vi "485 comm RT Driver VI.vi"(6 "Device Clock":string, 9 "Device Inputs FIFO":refnum<k33>, 10 "Device Outputs FIFO":refnum<k33>, 11 "Device Reference":T1 format="%.0x") -> ()   [LabVIEW 2015, in "485 comm Custom Device.lvlib"]
uses:
  485 comm Custom Device.lvlib
  <vilib>/NI Veristand/Custom Device API/Custom Device Item Ref.ctl
  <vilib>/NI Veristand/Custom Device API/Custom Device Channel Type.ctl
  Serial - Settings.ctl
  <vilib>/NI Veristand/Custom Device API/Message Response (String).ctl
  <vilib>/NI Veristand/Custom Device API/Message Response (Byte Array).ctl
  <vilib>/NI Veristand/Custom Device API/Get Item Property (Variant).vi
  <vilib>/NI Veristand/Custom Device API/Get Item Property (String).vi
  <vilib>/NI Veristand/Custom Device API/Get Item Property (U16).vi
  <vilib>/NI Veristand/Custom Device API/Get Item Property (U32).vi
  <vilib>/Instr/_visa.llb/VISA Configure Serial Port (Instr).vi
  <vilib>/NI Veristand/Custom Device API/Get Item Property (Boolean).vi
  <vilib>/NI Veristand/Custom Device API/Custom Device API.lvlib
  <vilib>/NI VeriStand/Custom Device Tools/Custom Device Utility Library/Custom Device Utility Library.lvlib
panel:
  in  "Initialization Status Notifier":refnum<notifier>
  in  "Status Notifier":refnum<notifier>
  # "Custom Device Template\nv1.0"
  # "Use this template as a starting point for creating a custom device code module. The input controls shown here are specially named controls that the system will use to provide the device loop with data. The controls are not required for the device loop to run. For instance, if the device doesn't produce any output data, then you don't need the Device Outputs FIFO control. If you do use these controls, however, they need to have these exact names to be functional."
  # "The optional status notifier element is used to notify the RT engine of the last state of the custom device, and to indicate the device has completed execution. If this control is not used, a default No Error value is returned to the system when the device finishes execution.\n\nNote: This error state is not checked until the system shuts down. Use an output status channel to send more immediate status values to the system."
  # "This optional input can be used to send the VeriStand Engine the final status of the custom device initalization process. If this control exists on the custom device front panel, the VeriStand Engine will wait for a status update before starting up. If the custom device reports an error, that will abort the execution of the current configuration in the VeriStand Engine.\n\nThis control can be deleted if the custom device does not need to send the initialization status update."
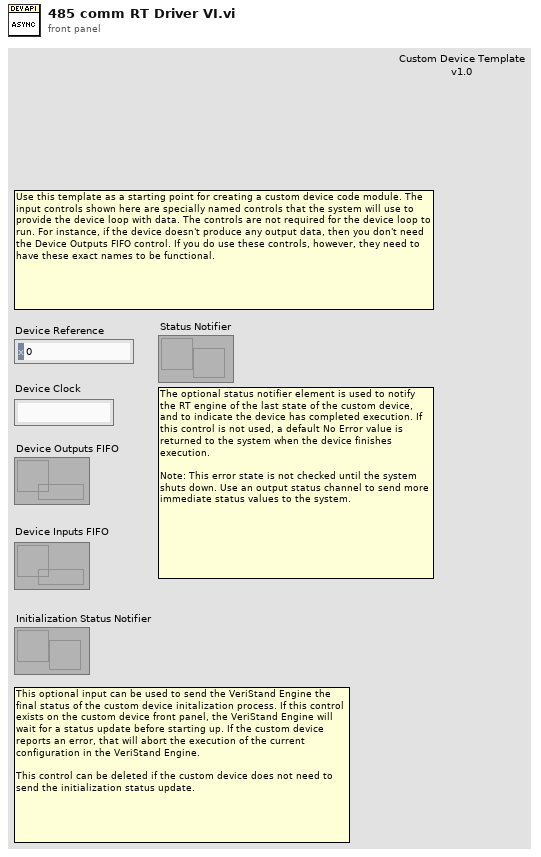
[diagram p1: front panel]
types:
  T1 = typedef "Custom Device API.lvlib/Custom Device Item Ref.ctl" = u64
  T2 = typedef "485 comm Custom Device.lvlib/Serial - Settings.ctl" = cluster{"baud rate":u32, "data bits":u16, "parity":enum16{"None", "Odd", "Even", "Mark", "Space"}, "stop bits":u16, "flow control":u16}
  T3 = typedef "Custom Device API.lvlib/Custom Device Channel Type.ctl" = enum16{"Input", "Output"}
  T4 = typedef "Custom Device API.lvlib/Custom Device Engine Event Ref.ctl" = refnum<event-registration>
  T5 = typedef "Custom Device API.lvlib/Message Response (String).ctl" = cluster{"Response":string, "Error":errorcluster}
  T6 = typedef "Custom Device API.lvlib/Message Response (Byte Array).ctl" = cluster{"Response":u8[], "Error":errorcluster}
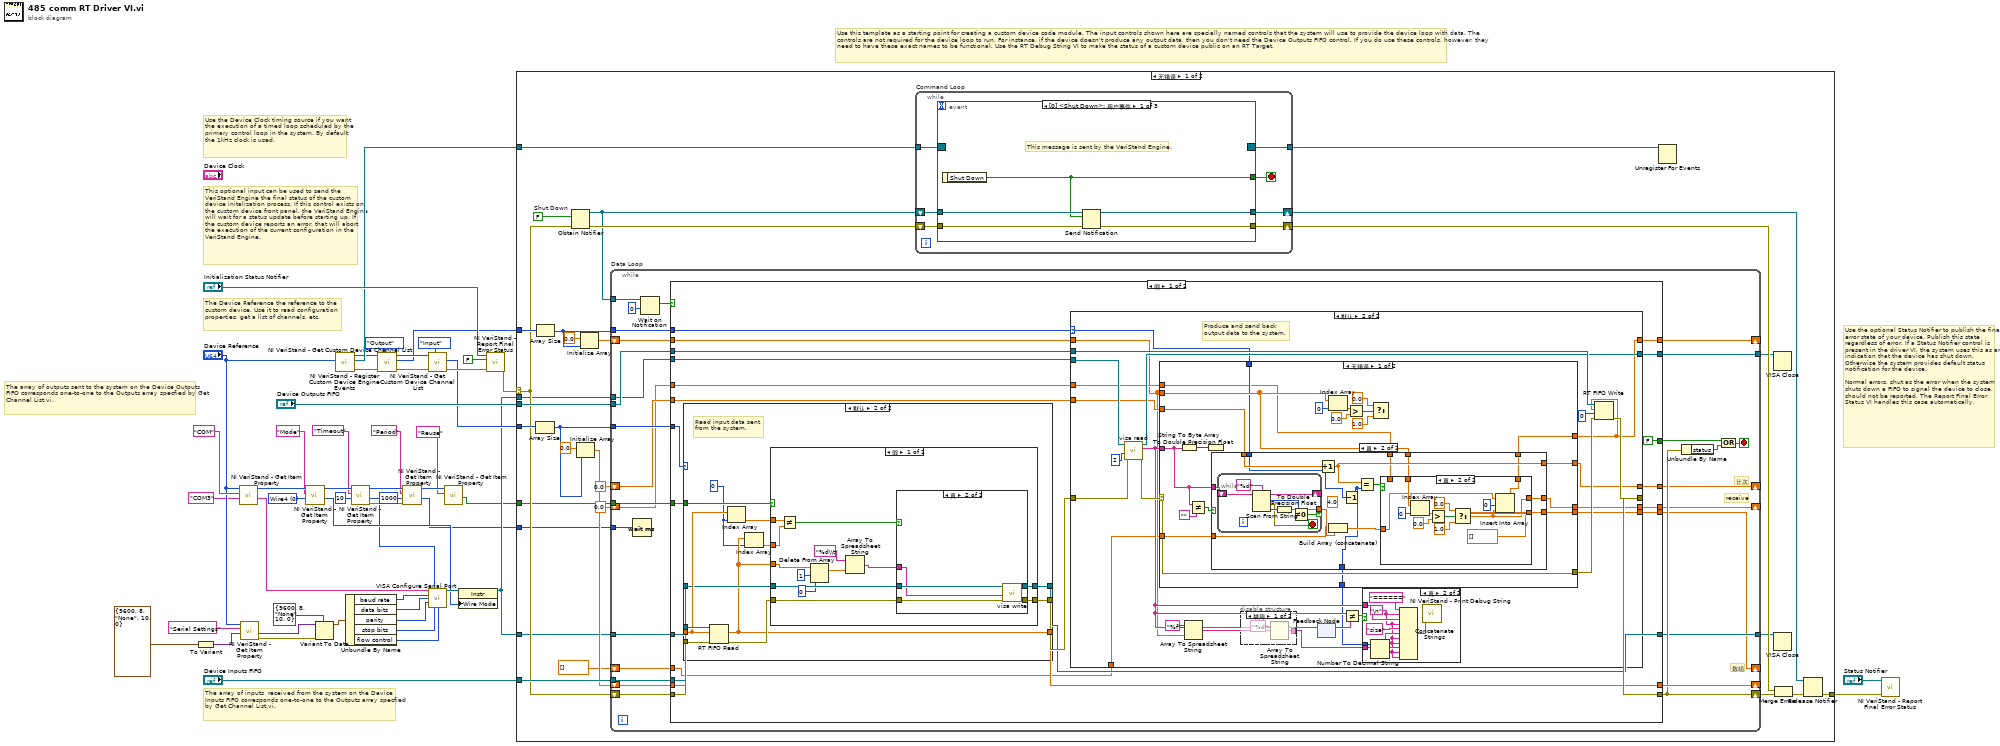
[diagram p0: block diagram]
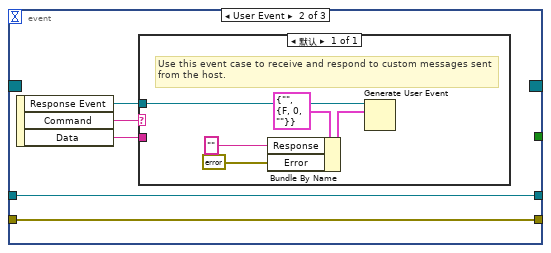
[diagram p2: hidden frame]
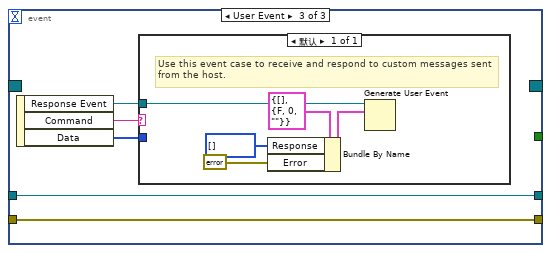
[diagram p3: hidden frame]
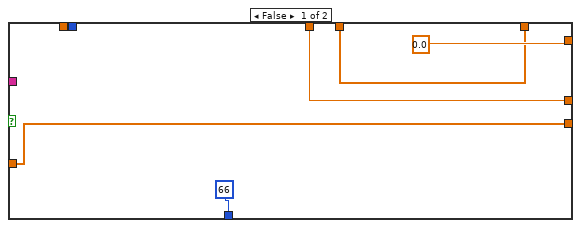
[diagram p7: hidden frame]
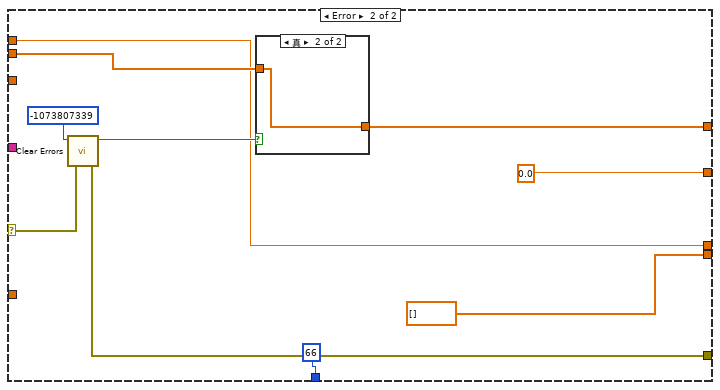
[diagram p9: hidden frame]
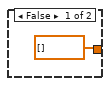
[diagram p10: hidden frame]
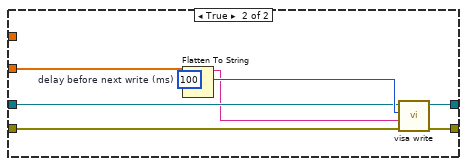
[diagram p13: hidden frame]
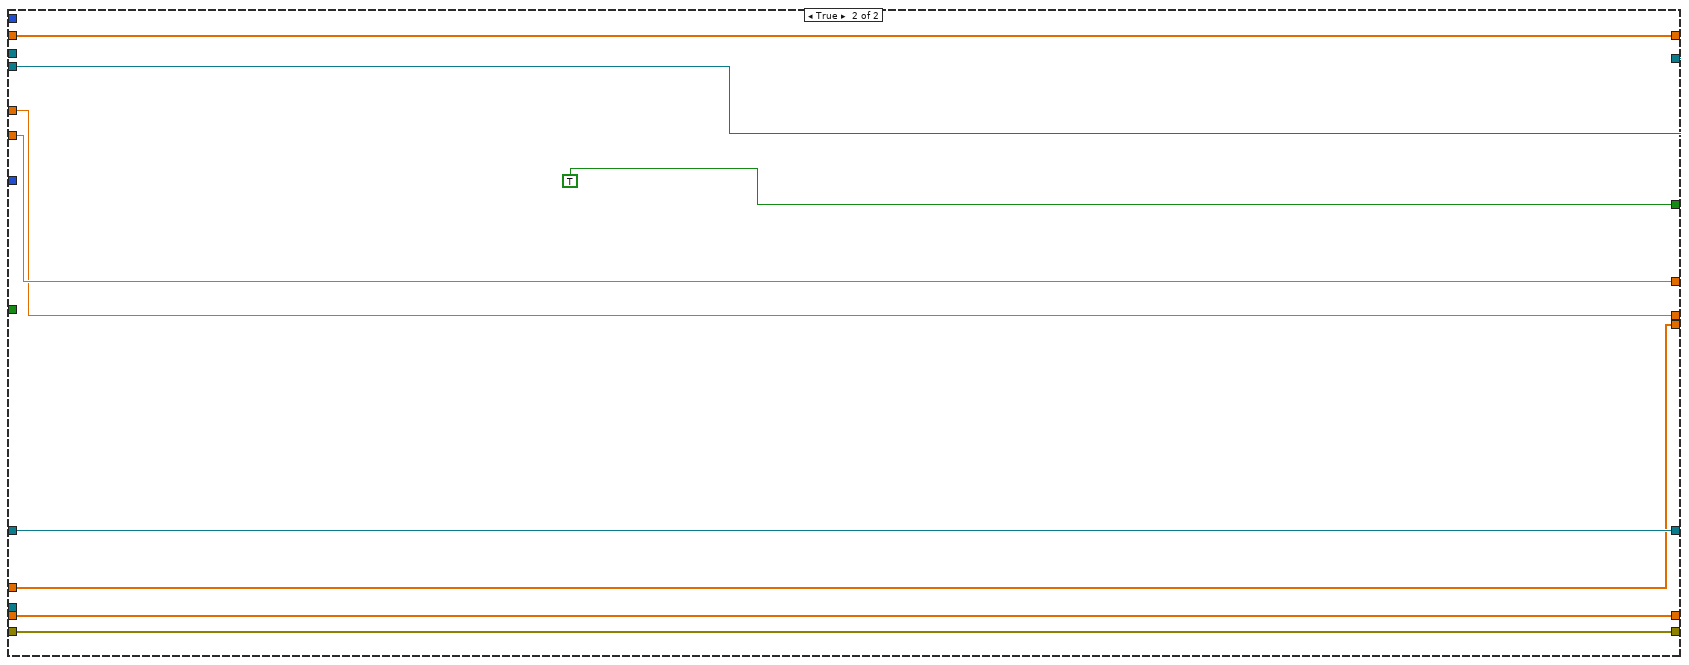
[diagram p14: hidden frame]
diagram:
  w14 = u16 0 items=["Wire4", "Wire2-EchoDTR", "Wire2-CtrlDTR", "Wire2-Auto"] ("RS-485 Transceiver Mode 2")
  # "This optional input can be used to send the VeriStand Engine the final status of the custom device initalization process. If this control exists on the custom device front panel, the VeriStand Engine will wait for a status update before starting up. If the custom device reports an error, that will abort the execution of the current configuration in the VeriStand Engine."
  # "The array of inputs  received from the system on the Device Inputs FIFO corresponds one-to-one to the Outputs array specfied by Get Channel List.vi."
  # "Use the optional Status Notifier to publish the final error state of your device. Publish this state regardless of error. If a Status Notifier control is present in the driver VI, the system uses this as an indication that the device has shut down. Otherwise the system provides default status notification for the device.\n\nNormal errors, shut as the error when the system shuts down a FIFO to signal the device to close, should not be reported. The Report Final Error Status VI handles this case automatically."
  # "The array of outputs sent to the system on the Device Outputs FIFO corresponds one-to-one to the Outputs array specfied by Get Channel List.vi."
  # "The Device Reference the reference to the custom device. Use it to read configuration properties, get a list of channels, etc."
  # "Use the Device Clock timing source if you want the execution of a timed loop scheduled by the primary control loop in the system. By default the 1kHz clock is used."
  # "Use this template as a starting point for creating a custom device code module. The input controls shown here are specially named controls that the system will use to provide the device loop with data. The controls are not required for the device loop to run. For instance, if the device doesn't produce any output data, then you don't need the Device Outputs FIFO control. If you do use these controls, however, they need to have these exact names to be functional. Use the RT Debug String VI to make the status of a custom device public on an RT Target."
  n1 = To Variant(anything=T2 {"baud rate"=9600, "data bits"=8, "parity"=enum."None", "stop bits"=10, "flow control"=0} ("Serial Settings")) -> (Variant=w27:variant)
  n2 = call-poly <vilib>:"NI VeriStand - Get Item Property.vi"("Default Value"="COM3", "Property Name"="COM", "Item Ref in"="Device Reference") -> ("Value"=w19:string, "Item Ref out"=w16:T1)  [unwired: 5 in, 2 out]
  n3 = call-poly <vilib>:"NI VeriStand - Get Item Property.vi"("Default Value"=w27, "Property Name"="Serial Settings", "Item Ref in"="Device Reference") -> ("error out"=w29:errorcluster, "Value"=w30:variant)  [unwired: 5 in, 2 out]
  n4 = call-poly <vilib>:"NI VeriStand - Get Item Property.vi"("Default Value"=w14, "Property Name"="Mode", "Item Ref in"=w16) -> ("Value"=w10:u16, "Item Ref out"=w13:T1)  [unwired: 5 in, 2 out]
  n5 = Variant To Data(error in=w29, type=T2 {"baud rate"=9600, "data bits"=8, "parity"=enum."None", "stop bits"=10, "flow control"=0} ("Serial Settings"), Variant=w30) -> (data=w28:T2)  [unwired: 1 out]
  n6 = call <vilib>:"NI VeriStand - Register Custom Device Engine Events.vi"("Device Ref in"="Device Reference") -> ("error out"=w51:errorcluster, "Custom Device Engine Event Ref"=w39:T4, "Device Ref out"=w37:T1)  [unwired: 8 in]
  n7 = Unbundle By Name(w28) -> ("baud rate"=w24:u32, "data bits"=w23:u16, "parity"=w22:enum16{"None", "Odd", "Even", "Mark", "Space"}, "stop bits"=w21:u16, "flow control"=w20:u16)
  n8 = call-poly <vilib>:"NI VeriStand - Get Item Property.vi"("Default Value"=u32 10, "Property Name"="Timeout", "Item Ref in"=w13) -> ("error out"=w9:errorcluster, "Value"=w8:u32, "Item Ref out"=w7:T1)  [unwired: 5 in, 1 out]
  n9 = call <vilib>:"NI VeriStand - Get Custom Device Channel List.vi"("Channel Type"=Custom_Device_Channel_Type."Output", "error in (no error)"=w51, "Device Ref in"=w37) -> ("error out"=w44:errorcluster, "Specified Channel Ref List"=w41:T1[], "Device Ref out"=w45:T1)  [unwired: 6 out]
  n10 = call-poly <vilib>:"NI VeriStand - Get Item Property.vi"("error in (no error)"=w9, "Default Value"=u32 1000, "Property Name"="Period", "Item Ref in"=w7) -> ("Value"=w4:u32, "Item Ref out"=w3:T1)  [unwired: 4 in, 2 out]
  n11 = call <vilib>:"NI VeriStand - Get Custom Device Channel List.vi"("Channel Type"=Custom_Device_Channel_Type."Input", "error in (no error)"=w44, "Device Ref in"=w45) -> ("error out"=w50:errorcluster, "Specified Channel Ref List"=w42:T1[])  [unwired: 7 out]
  n12 = call-poly "VISA Configure Serial Port"("VISA resource name"=w19, "timeout (10sec)"=w8, "baud rate (9600)"=w24, "data bits (8)"=w23, "parity (0:none)"=w22, "stop bits (10: 1 bit)"=w21, "flow control (0:none)"=w20) -> ("VISA resource name out"=w18:refnum<visa-resource-name>)  [unwired: 2 in, 6 out]
  n13 = call-poly <vilib>:"NI VeriStand - Get Item Property.vi"("Property Name"="Reuse", "Item Ref in"=w3) -> ("Value"=w1:bool)  [unwired: 6 in, 3 out]
  n14 = property class="Instr"(reference=w18, "Wire Mode"=w10) -> (reference out=w17:refnum<visa-resource-name>)  [unwired: 1 in, 1 out]
  n15 = call <vilib>:"NI VeriStand - Report Final Error Status.vi"("error in (no error)"=w50, "Filter FIFO & Shutdown Errors (T)"=FALSE ("Filter FIFO Errors (T)"), "Status Notifier"="Initialization Status Notifier") -> ("error out"=w36:errorcluster)  [unwired: 8 out]
  n16 = case shown="无错误" w36 {
    selector: w36 -> [w63 w331]
    tunnel: "Device Outputs FIFO" -> [w80 _]
    tunnel: "Device Inputs FIFO" -> [w79 _]
    tunnel: w42 -> [w73 _]
    tunnel: w41 -> [w72 _]
    tunnel: w39 -> [w70 _]
    tunnel: [w68 w331] -> w38
    tunnel: w17 -> [w60 _]
    tunnel: w17 -> [w58 _]
    tunnel: w4 -> [w56 _]
    tunnel: w1 -> [w55 _]
    frame No Error {
      w69 = FALSE  # Shut Down
      n17 = Array Size(array=w73) -> (size(s)=w71:i32)
      n18 = Array Size(array=w72) -> (size(s)=w74:i32)
      n19 = Obtain Notifier(notification data type=w69, error in (no error)=w63) -> (notifier out=w66:refnum<notifier>, error out=w81:errorcluster)  [unwired: 2 in, 1 out]
      n20 = Initialize Array(0.0 ("element"), w71) -> (w75:dbl[])
      n21 = Initialize Array(0.0 ("element"), w74) -> (w76:dbl[])
      n22 = while "Data Loop" {
        shift-right: [w139] -> _
        shift-left: w75 -> [w140]
        shift-right: [w131] -> w64
        shift-left: w63 -> [w141]
        shift-right: [w137] -> _
        shift-left: w76 -> [w138]
        tunnel: w74 -> [w134]
        tunnel: w80 -> [w136]
        tunnel: w79 -> [w135]
        tunnel: w71 -> [w133]
        tunnel: w66 -> [w130]
        tunnel: w60 -> [w125]
        tunnel: [w124] -> w59
        tunnel: w58 -> [w123]
        tunnel: [w122] -> w57
        tunnel: w56 -> [w121]
        tunnel: w55 -> [w120]
        shift-right: [w119] -> _
        shift-left: 0.0 -> [w118]
        shift-right: [w116] -> _
        shift-left: dbl[] [] -> [w117]
        shift-right: [w115] -> _
        shift-left: 0.0 ("f") -> [w114]
        stop <- w126 stop-if-true
        # "receive"
        # "数组"
        # "计次"
        n23 = Wait (ms) ("等待(ms)")(milliseconds to wait=w121) -> ()  [unwired: 1 out]
        n24 = Wait on Notification(notifier=w130, timeout in ms (-1)=0) -> (notification=w129:bool)  [unwired: 2 in, 3 out]
        n25 = case shown="假" w129 {
          tunnel: w141 -> [w164 w329]
          tunnel: w140 -> [w163 w330]
          tunnel: [w150 w330] -> w139
          tunnel: w138 -> [w155 w328]
          tunnel: [w162 w328] -> w137
          tunnel: w136 -> [w161 _]
          tunnel: w135 -> [w160 _]
          tunnel: w134 -> [w159 _]
          tunnel: w133 -> [w158 _]
          tunnel: [w156 w329] -> w131
          tunnel: [FALSE TRUE] -> w127
          tunnel: w125 -> [w154 w326]
          tunnel: [w153 w326] -> w124
          tunnel: w123 -> [w152 w325]
          tunnel: [w151 w325] -> w122
          tunnel: w120 -> [w148 _]
          tunnel: [w147 w324] -> w119
          tunnel: w118 -> [w146 w324]
          tunnel: w117 -> [w145 w323]
          tunnel: [w144 w323] -> w116
          tunnel: [w143 w322] -> w115
          tunnel: w114 -> [w142 w322]
          frame False {
            n26 = case shown="默认" w158 {
              tunnel: w160 -> [_ w294]
              tunnel: w163 -> [w282 w292]
              tunnel: [w282 w284] -> w150
              tunnel: [w281 w286] -> w157
              tunnel: w164 -> [w281 w293]
              tunnel: w152 -> [w280 w288]
              tunnel: [w280 w285] -> w151
              tunnel: w148 -> [_ w291]
              frame 0 {
                # "No inputs to read\nfrom system. Inputs FIFO not created in this case, so don't write to it."
              }
              frame Default {
                w283 = 0 ("索引")
                # "Read input data sent from the system."
                n27 = RT FIFO Read(0:w294, 1:w292, 3:w293) -> (9:w284:dbl[], 11:w287:errorcluster)  [unwired: 4 out]
                n28 = Index Array(array=w292, index=w283) -> (element=w289:dbl)
                n29 = Index Array(array=w284, index=w283) -> (element=w290:dbl)
                n30 = case shown="假" w291 {
                  tunnel: w290 -> [w302 _]
                  tunnel: w289 -> [w307 _]
                  tunnel: w288 -> [w305 w320]
                  tunnel: w287 -> [w306 w319]
                  tunnel: [w304 w318] -> w286
                  tunnel: [w303 w317] -> w285
                  tunnel: w284 -> [w298 w316]
                  frame False {
                    n31 = Not Equal?(x=w307, y=w302) -> (x != y?=w301:bool)
                    n32 = Delete From Array(array=w298, length=1 ("长度"), index=0 ("索引")) -> (array with subset deleted=w297:dbl[])  [unwired: 1 out]
                    n33 = Array To Spreadsheet String(array=w297, 3:"%d\\t" ("格式字符串")) -> (spreadsheet string=w295:string)  [unwired: 1 in]
                    n34 = case shown="真" w301 {
                      tunnel: w306 -> [w308 w314]
                      tunnel: w305 -> [w309 w313]
                      tunnel: [w308 w312] -> w304
                      tunnel: [w309 w311] -> w303
                      tunnel: w295 -> [_ w310]
                      frame False {
                      }
                      frame True {
                        n35 = call "visa write.vi"("error in (no error)"=w314, "input"=w310, "VISA resource name"=w313) -> ("error out"=w312:errorcluster, "VISA resource name out"=w311:refnum<visa-resource-name>)  [unwired: 7 in]
                      }
                    }
                  }
                  frame True {
                    w321 = u32 100  # delay before next write (ms)
                    n36 = Flatten To String(anything=w316) -> (data string=w315:string)  [unwired: 3 in, 2 out]
                    n37 = call "visa write.vi"("error in (no error)"=w319, "input"=w315, "delay before next writte (ms)"=w321, "VISA resource name"=w320) -> ("error out"=w318:errorcluster, "VISA resource name out"=w317:refnum<visa-resource-name>)  [unwired: 6 in]
                  }
                }
              }
            }
            n38 = case shown="默认" w159 {
              selector: w159 -> [_ w177]
              tunnel: w161 -> [_ w194]
              tunnel: w155 -> [w170 w173]
              tunnel: w157 -> [w169 w189]
              tunnel: [w169 w193] -> w156
              tunnel: [w170 w184] -> w162
              tunnel: w154 -> [w168 w191]
              tunnel: [w168 w190] -> w153
              tunnel: [w167 w181] -> w147
              tunnel: w146 -> [w167 w180]
              tunnel: w145 -> [w166 w179]
              tunnel: [w166 w178] -> w144
              tunnel: [w165 w175] -> w143
              tunnel: w142 -> [w165 w174]
              frame 0 {
                # "No outputs to write to system. The Device Outputs FIFO is never created in this case, so don't write to it."
              }
              frame Default {
                # "Produce and send back output data to the system."
                n39 = call "visa read.vi"("error in"=w189, "字节总数"=u32 2, "VISA resource name in"=w191) -> ("error out"=w188:errorcluster, "String of array"=w182:string, "VISA resource name out"=w190:refnum<visa-resource-name>)  [unwired: 5 in, 1 out]
                n40 = case shown="无错误" w188 {
                  selector: w188 -> [w225 w277]
                  tunnel: [w205 w273] -> w184
                  tunnel: [w225 w274] -> w187
                  tunnel: w173 -> [w211 w272]
                  tunnel: w182 -> [w217 _]
                  tunnel: [w215 0.0] -> w181
                  tunnel: w180 -> [w214 _]
                  tunnel: w179 -> [w213 _]
                  tunnel: [w212 dbl[] []] -> w178
                  tunnel: w177 -> [w210 _]
                  tunnel: [w209 66] -> w176
                  tunnel: [w207 w268] -> w175
                  tunnel: w174 -> [w206 w268]
                  frame No Error {
                    n41 = String To Byte Array(string=w217) -> (unsigned byte array=w224:u8[])
                    n42 = Not Equal?(x=w217, y="") -> (x != y?=w216:bool)
                    n43 = To Double Precision Float(number=w224) -> ()  [unwired: 1 out]
                    n44 = case shown="真" w216 {
                      tunnel: w217 -> [_ w244]
                      tunnel: [0.0 w240] -> w215
                      tunnel: w214 -> [_ w243]
                      tunnel: w213 -> [w229 w241]
                      tunnel: [w229 w237] -> w212
                      tunnel: w211 -> [w226 w236]
                      tunnel: w210 -> [_ w235]
                      tunnel: [66 w234] -> w209
                      tunnel: [w227 w233] -> w207
                      tunnel: w206 -> [w227 w232]
                      tunnel: [w226 w231] -> w205
                      frame False {
                      }
                      frame True {
                        (unwired) 4.0 ("y")
                        n45 = while {
                          shift-right: [w265] -> _
                          shift-left: w244 -> [w267]
                          tunnel: [w263] -> w242 if=w261
                          stop <- w262 stop-if-true
                          n46 = Scan From String(format string="%d" ("格式字符串"), input string=w267) -> (remaining string=w265:string, offset past scan=w260:u32, error out=w262:errorcluster, output 1=w264:i32)  [unwired: 3 in]
                          n47 = To Double Precision Float(number=w264) -> (double precision float=w263:dbl)
                          n48 = Not Equal To 0?(x=w260) -> (x != 0?=w261:bool)
                        }
                        n49 = Increment(x=w243) -> (x+1=w240:dbl)
                        n50 = Build Array (concatenate)(w241, w242) -> (w238:dbl[])
                        n51 = Decrement(x=w235) -> (x-1=w234:i32)
                        n52 = Equal?(x=w240, y=w234) -> (x = y?=w239:bool)
                        n53 = case shown="真" w239 {
                          tunnel: w238 -> [w247 w250]
                          tunnel: [w247 dbl[] []] -> w237
                          tunnel: w236 -> [w245 w252]
                          tunnel: [w246 w248] -> w233
                          tunnel: w232 -> [w246 _]
                          tunnel: [w245 w249] -> w231
                          frame False {
                          }
                          frame True {
                            n54 = Index Array(array=w252, index=0 ("索引")) -> (element=w258:dbl)
                            n55 = Greater?(x=w258, y=0.0) -> (0:w256:bool)
                            n56 = Select(t=0.0, s=w256, f=1.0) -> (s? t:f=w248:dbl)
                            n57 = Insert Into Array(array=w250, index=0 ("索引"), new element=w248) -> (w249:dbl[])
                          }
                        }
                      }
                    }
                    n58 = Index Array(array=w211, index=0 ("索引")) -> (element=w223:dbl)
                    n59 = Greater?(x=w223, y=0.0) -> (0:w221:bool)
                    n60 = Select(t=0.0, s=w221, f=1.0) -> ()  [unwired: 1 out]
                  }
                  frame Error {
                    n61 = call <vilib>:"Clear Errors.vi"("error in (no error)"=w277, "specific error code to clear (0: all)"=-1073807339 ("y")) -> ("error out"=w274:errorcluster, "specific error cleared?"=w275:bool)  [unwired: 4 in]
                    n62 = case shown="真" w275 {
                      tunnel: [dbl[] [] w279] -> w273
                      tunnel: w272 -> [_ w279]
                      frame False {
                      }
                      frame True {
                      }
                    }
                  }
                }
                n63 = Array To Spreadsheet String(array=w173, 3:"%f" ("格式字符串")) -> (spreadsheet string=w171:string)  [unwired: 1 in]
                n64 = disable-structure shown="禁用" {
                  disable-tunnel: [w196 _] -> _
                  frame Disabled {
                    n65 = Array To Spreadsheet String(3:"%d" ("格式字符串")) -> (spreadsheet string=w196:string)  [unwired: 2 in]
                  }
                  frame Enabled {
                  }
                }
                n66 = feedback-in #1(w182) -> ()
                n67 = feedback #1() -> (w186:string)  [unwired: 1 in]
                n68 = Not Equal?(x=w182, y=w186) -> (x != y?=w185:bool)
                n69 = case shown="真" w185 {
                  tunnel: w182 -> [_ w203]
                  tunnel: w176 -> [_ w199]
                  tunnel: w171 -> [_ w198]
                  frame False {
                  }
                  frame True {
                    w197 = "\n"
                    n70 = Number To Decimal String(number=w199) -> (decimal integer string=w200:string)  [unwired: 1 in]
                    n71 = Concatenate Strings("======" ("字符串"), w197, w203, w197, "size" ("字符串"), w200, w197, w197, w198, w197, w197) -> (w204:string)
                    n72 = call <vilib>:"NI VeriStand - Print Debug String.vi"("Message"=w204) -> ()  [unwired: 10 in, 1 out]
                  }
                }
                n73 = RT FIFO Write(0:w194, 1:w184, 2:0 ("timeout in ms (0)"), 3:w187) -> (11:w193:errorcluster)  [unwired: 1 in, 3 out]
              }
            }
          }
          frame True {
          }
        }
        n74 = Unbundle By Name(w131) -> ("status"=w128:bool)
        n75 = Compound Arithmetic op=OR(w127, w128) -> (w126:bool)
      }
      n76 = while "Command Loop" {
        tunnel: w70 -> [w88]
        tunnel: [w87] -> w67
        shift-right: [w84] -> w65
        shift-left: w66 -> [w85]
        shift-right: [w82] -> w61
        shift-left: w81 -> [w83]
        stop <- w86 stop-if-true
        n77 = event shown="[0] <Shut Down>: 用户事件" {
          selector: w88 -> [_ _ _]
          dyn-events: [_ _ _] -> w87
          timeout: _ -> [_ _ _]
          tunnel: [w91 _ _] -> w86
          tunnel: w85 -> [w92 w96 w106]
          tunnel: [w93 w96 w106] -> w84
          tunnel: w83 -> [w90 w94 w104]
          tunnel: [w89 w94 w104] -> w82
          event User Event {
            # "This message is sent by the VeriStand Engine."
            n78 = event-data() -> ("Shut Down"=w91:bool)  [unwired: 1 in]
            n79 = Send Notification(notification=w91, notifier=w92, error in (no error)=w90) -> (notifier out=w93:refnum<notifier>, error out=w89:errorcluster)
          }
          event User Event {
            n80 = event-data() -> ("Response Event"=w95:refnum<user-event>, "Command"=w98:string, "Data"=w97:string)  [unwired: 1 in]
            n81 = case shown="默认" w98 {
              tunnel: w97 -> [_]
              tunnel: w95 -> [w103]
              frame 默认 {
                # "Use this event case to receive and respond to custom messages sent from the host."
                n82 = Bundle By Name(cluster=T5 {"Response"="", "Error"={"status"=FALSE, "code"=0, "source"=""}} ("event data"), "Response"="", "Error"=errorcluster {"status"=FALSE, "code"=0, "source"=""}) -> (w101:T5)
                n83 = Generate User Event(user event=w103, event data cluster=w101) -> ()  [unwired: 2 in, 2 out]
              }
            }
          }
          event User Event {
            n84 = event-data() -> ("Response Event"=w105:refnum<user-event>, "Command"=w108:string, "Data"=w107:u8[])  [unwired: 1 in]
            n85 = case shown="默认" w108 {
              tunnel: w107 -> [_]
              tunnel: w105 -> [w113]
              frame 默认 {
                # "Use this event case to receive and respond to custom messages sent from the host."
                n86 = Bundle By Name(cluster=T6 {"Response"=[], "Error"={"status"=FALSE, "code"=0, "source"=""}} ("event data"), "Response"=u8[] [], "Error"=errorcluster {"status"=FALSE, "code"=0, "source"=""}) -> (w110:T6)
                n87 = Generate User Event(user event=w113, event data cluster=w110) -> ()  [unwired: 2 in, 2 out]
              }
            }
          }
        }
      }
      n88 = Unregister For Events(event registration refnum=w67) -> ()  [unwired: 1 in, 1 out]
      n89 = VISA Close(VISA resource name=w59) -> ()  [unwired: 1 in, 1 out]
      n90 = VISA Close(VISA resource name=w57) -> ()  [unwired: 1 in, 1 out]
      n91 = Merge Errors(w61, w64) -> (w62:errorcluster)
      n92 = Release Notifier(notifier=w65, error in (no error)=w62) -> (error out=w68:errorcluster)  [unwired: 1 in, 2 out]
    }
    frame Error {
    }
  }
  n93 = call <vilib>:"NI VeriStand - Report Final Error Status.vi"("error in (no error)"=w38, "Status Notifier"="Status Notifier") -> ()  [unwired: 1 in, 9 out]
